vi "HAPS_LoadTable_SetBeam.vi"() -> ()   [LabVIEW 2023, in "HAPS.lvlib"]
uses:
  HAPS.lvlib
  set_ele.ctl
  HAPS_MCU_ELE_Func.ctl
  <vilib>/Utility/file.llb/Read Delimited Spreadsheet (string).vi
panel:
  in  "VISA resource name":refnum<visa-resource-name>="COM1"
  out "ele phase":i32
  out "ele gain":i32
  out "channel":i32
  out "chain ID":i32
  out "group":i32
  out "array id":i32
  out "Remaining quantity":i32
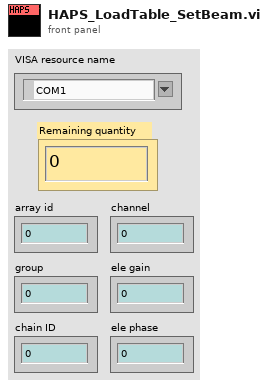
[diagram p1: front panel]
types:
  T1 = typedef "HAPS.lvlib/set_ele.ctl" = cluster{"ch":i32, "chain_id":i32, "group":i32, "array_id":i32, "ele_phase":i32, "ele_gain":i32, "com_gain":i32, "pd_range":i32}
  T2 = typedef "HAPS.lvlib/HAPS_MCU_ELE_Func.ctl" = enum16{"array_init", "set_com_gain", "set_ch_gain_phase", "set_pd_range", "get_preamp_temp", "get_bfic_temp", "get_tx_pd", "ch_on", "ch_on_2", "ch_ctrl_all", "array_ctrl_src"}
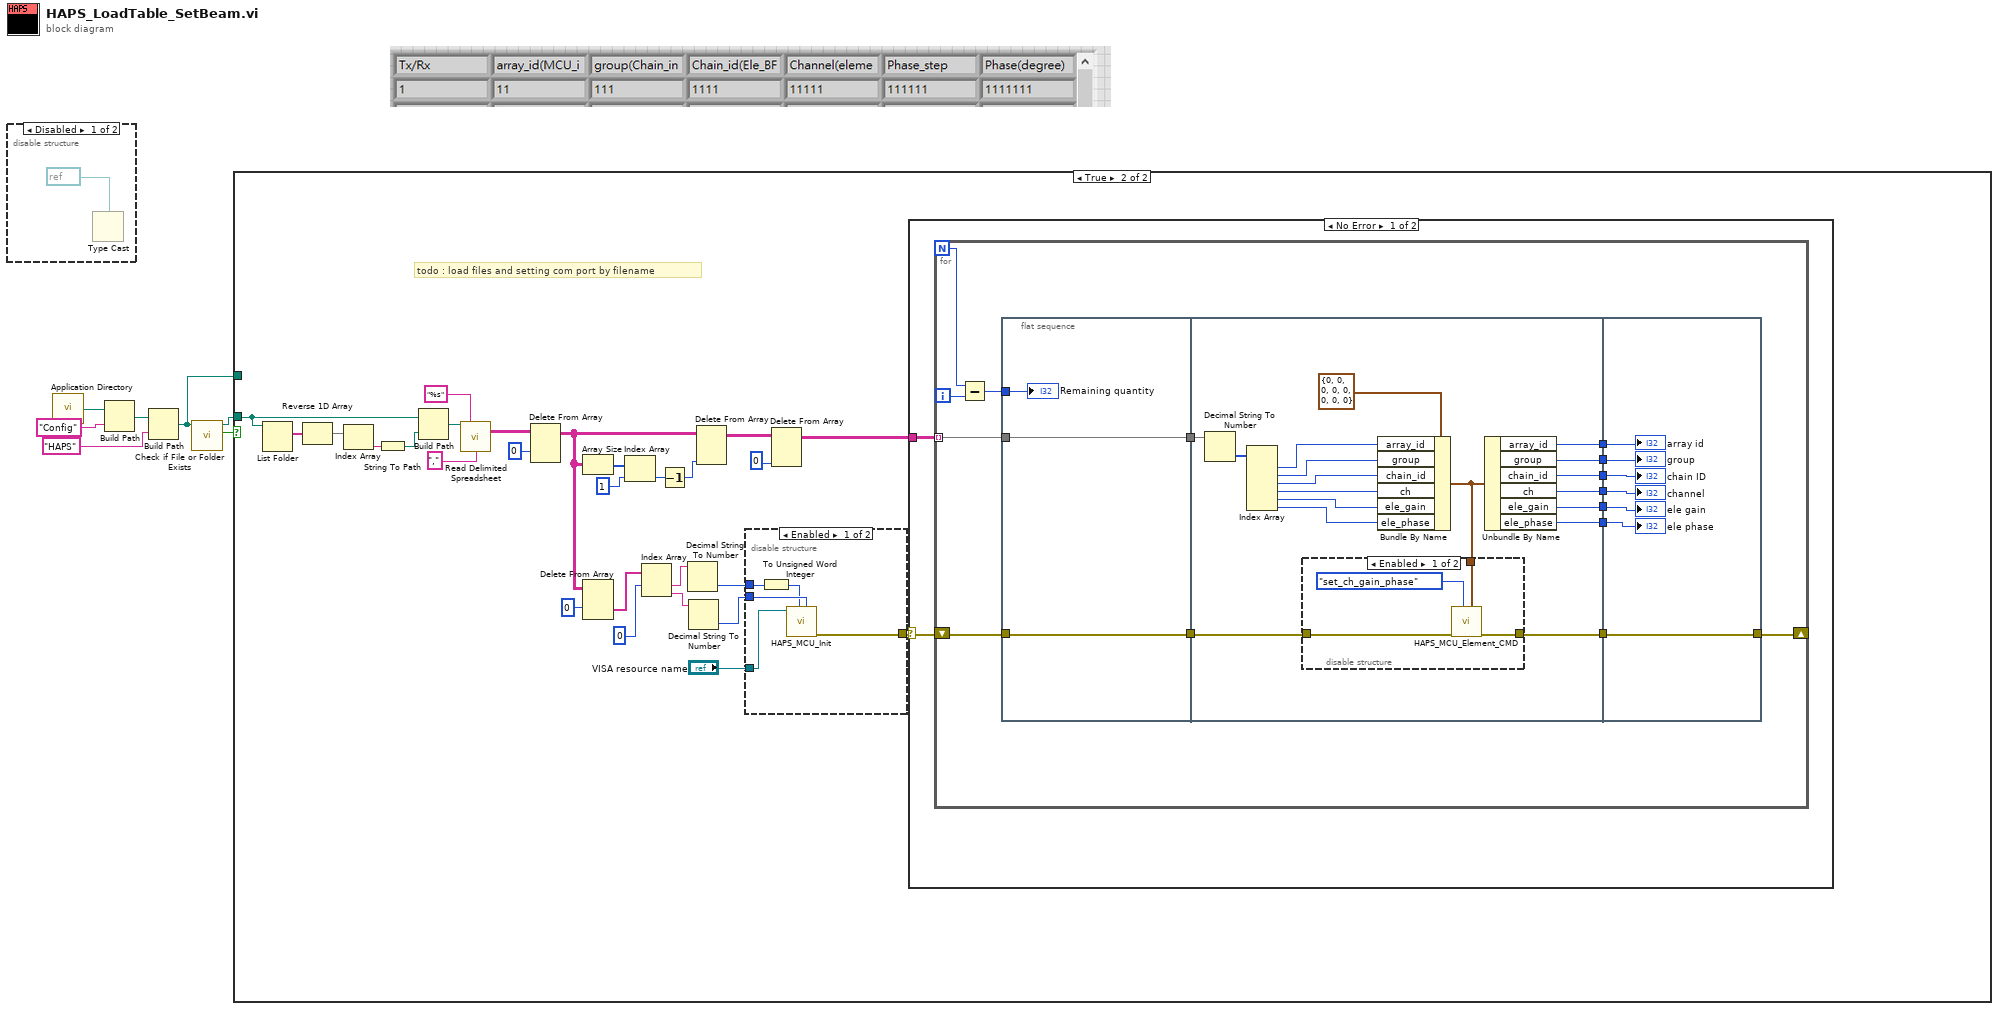
[diagram p0: block diagram]
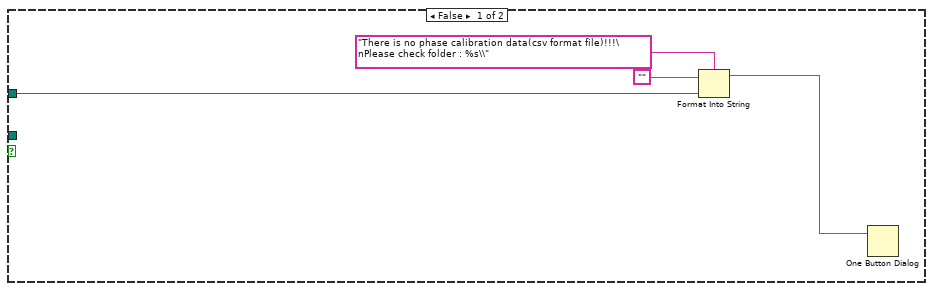
[diagram p3: hidden frame]
diagram:
  n1 = disable-structure shown="Disabled" {
    frame Disabled {
      n2 = Type Cast(type=refnum<visa-resource-name> refnum ("VISA resource name")) -> ()  [unwired: 1 in, 1 out]
    }
    frame Enabled {
    }
  }
  n3 = call <vilib>:"Application Directory.vi"() -> ("Application Directory"=w6:path)
  n4 = Build Path(base path=w6, name or relative path="Config") -> (appended path=w4:path)
  n5 = Build Path(base path=w4, name or relative path="HAPS") -> (appended path=w1:path)
  n6 = call <vilib>:"Check if File or Folder Exists.vi"("path"=w1) -> ("file or folder exists?"=w3:bool, "dup path"=w2:path)  [unwired: 8 in, 1 out]
  n7 = case shown="True" w3 {
    tunnel: w2 -> [_ w35]
    tunnel: w1 -> [w12 _]
    frame False {
      n8 = Format Into String(format string="There is no phase calibration data(csv format file)!!!\nPlease check folder : %s\\" ("message"), initial string="", w12) -> (resulting string=w9:string)  [unwired: 1 in, 1 out]
      n9 = One Button Dialog(message=w9) -> ()  [unwired: 1 in, 1 out]
    }
    frame True {
      # "todo : load files and setting com port by filename"
      n10 = List Folder(path=w35) -> (filenames=w39:string[])  [unwired: 3 in, 3 out]
      n11 = Reverse 1D Array(array=w39) -> (reversed array=w38:string[])
      n12 = Index Array(array=w38) -> (element=w37:string)  [unwired: 1 in]
      n13 = String To Path(string=w37) -> (path=w36:path)
      n14 = Build Path(base path=w35, name or relative path=w36) -> (appended path=w34:path)
      n15 = call-poly <vilib>:"Read Delimited Spreadsheet.vi"("file path (dialog if empty)"=w34, "format (%s)"="%s" ("format (%.3f)"), "delimiter (\\t)"="," ("delimiter (\\t)")) -> ("all rows"=w31:string[][])  [unwired: 7 in, 5 out]
      n16 = Delete From Array(array=w31, index (row)=0) -> (array with subset deleted=w20:string[][])  [unwired: 2 in, 1 out]
      n17 = Array Size(array=w20) -> (size(s)=w29:i32[])
      n18 = Delete From Array(array=w20, index (row)=0) -> (deleted portion=w19:string[])  [unwired: 2 in, 1 out]
      n19 = Index Array(array=w29, index=1) -> (element=w26:i32)
      n20 = Index Array(array=w19, index #1=0 ("index")) -> (element #1=w18:string, element #2=w17:string)  [unwired: 1 in]
      n21 = Decrement(x=w26) -> (x-1=w28:i32)
      n22 = Decimal String To Number(string=w18) -> (number=w14:i32)  [unwired: 2 in, 1 out]
      n23 = Decimal String To Number(string=w17) -> (number=w13:i32)  [unwired: 2 in, 1 out]
      n24 = Delete From Array(array=w20, index (col)=w28) -> (array with subset deleted=w24:string[][])  [unwired: 2 in, 1 out]
      n25 = disable-structure shown="Enabled" {
        disable-tunnel: [w44 _] -> w25
        disable-tunnel: w14 -> [w43 _]
        disable-tunnel: w13 -> [w42 _]
        disable-tunnel: "VISA resource name" -> [w41 _]
        frame Enabled {
          n26 = To Unsigned Word Integer(number=w43) -> (unsigned 16bit integer=w40:u16)
          n27 = call "HAPS_MCU_Init.vi"("array_id"=w42, "Tx/Rx"=w40, "VISA resource name"=w41) -> ("error out"=w44:errorcluster)  [unwired: 8 in]
        }
        frame Disabled {
        }
      }
      n28 = Delete From Array(array=w24, index (col)=0 ("index (row)")) -> (array with subset deleted=w23:string[][])  [unwired: 2 in, 1 out]
      n29 = case shown="No Error" w25 {
        selector: w25 -> [w45 _]
        tunnel: w23 -> [w46 _]
        frame No Error {
          n30 = for {
            N -> [w55]
            tunnel: w46 -> [w61] mode=indexing
            shift-right: [w60] -> _
            shift-left: w45 -> [w59]
            i -> [w56]
            n31 = Subtract(x=w55, y=w56) -> (x-y=w54:i32)
            n32 = flat-sequence {
              tunnel: w59 -> [w63]
              tunnel: w61 -> [w64]
              tunnel: [w64] -> w58
              tunnel: [w63] -> w57
              tunnel: w54 -> [w62]
              tunnel: w58 -> [w82]
              tunnel: w57 -> [w79]
              tunnel: [w80] -> w53
              tunnel: [w70] -> w52
              tunnel: [w69] -> w51
              tunnel: [w68] -> w50
              tunnel: [w67] -> w49
              tunnel: [w66] -> w48
              tunnel: [w65] -> w47
              tunnel: [w94] -> w60
              tunnel: w53 -> [w94]
              tunnel: w52 -> [w93]
              tunnel: w51 -> [w92]
              tunnel: w50 -> [w91]
              tunnel: w49 -> [w90]
              tunnel: w48 -> [w89]
              tunnel: w47 -> [w88]
              frame #0 {
                "Remaining quantity" <- w62
              }
              frame #1 {
                n33 = Decimal String To Number(string=w82) -> (number=w81:i32[])  [unwired: 2 in, 1 out]
                n34 = Index Array(array=w81) -> (element #1=w77:i32, element #2=w76:i32, element #3=w75:i32, element #4=w74:i32, element #5=w73:i32, element #6=w72:i32)  [unwired: 6 in]
                n35 = Bundle By Name(cluster=T1 {"ch"=0, "chain_id"=0, "group"=0, "array_id"=0, "ele_phase"=0, "ele_gain"=0, "com_gain"=0, "pd_range"=0} ("set_ele"), "array_id"=w77, "group"=w76, "chain_id"=w75, "ch"=w74, "ele_gain"=w73, "ele_phase"=w72) -> (w71:T1)
                n36 = disable-structure shown="Enabled" {
                  disable-tunnel: [w86 w87] -> w80
                  disable-tunnel: w79 -> [w85 w87]
                  disable-tunnel: w71 -> [w83 _]
                  frame Enabled {
                    n37 = call "HAPS_MCU_Element_CMD.vi"("set_ele"=w83, "HAPS_MCU_ELE_Func."=HAPS_MCU_ELE_Func."set_ch_gain_phase", "error in"=w85) -> ("error out"=w86:errorcluster)  [unwired: 7 in, 1 out]
                  }
                  frame Disabled {
                  }
                }
                n38 = Unbundle By Name(w71) -> ("array_id"=w70:i32, "group"=w69:i32, "chain_id"=w68:i32, "ch"=w67:i32, "ele_gain"=w66:i32, "ele_phase"=w65:i32)
              }
              frame #2 {
                "group" <- w92
                "chain ID" <- w91
                "channel" <- w90
                "ele gain" <- w89
                "ele phase" <- w88
                "array id" <- w93
              }
            }
          }
        }
        frame Error {
        }
      }
    }
  }
